vi "Pre Launch Init.vi"(11 "UI in":refnum<class "UI.lvclass">) -> (0 "error out":errorcluster, 3 "UI out":refnum<class "UI.lvclass">)   [LabVIEW 2016, in "UI.lvlib" / "UI.lvclass"]
doc: "Creates user events for the UI actor which later can be used to receive messages"
uses:
  UI.lvclass
  <vilib>/vision/Image Controls.llb/IMAQ Image.ctl
  UI.lvclass/UI.ctl
  <vilib>/ActorFramework/Actor/Actor.lvclass
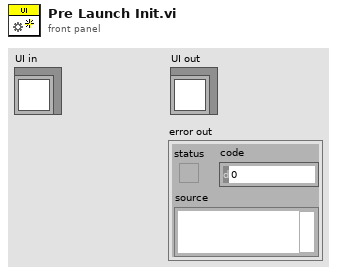
[diagram p1: front panel]
types:
  T1 = typedef "IMAQ Image.ctl" = refnum<image>
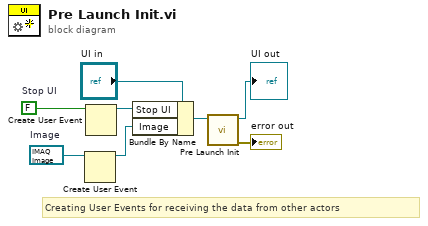
[diagram p0: block diagram]
diagram:
  w2 = T1 refnum  # Image
  w4 = FALSE  # Stop UI
  # "Creating User Events for receiving the data from other actors"
  n1 = Create User Event(user event datatype=w2) -> (user event=w1:refnum<user-event>)  [unwired: 1 in, 1 out]
  n2 = Create User Event(user event datatype=w4) -> (user event=w3:refnum<user-event>)  [unwired: 1 in, 1 out]
  n3 = Bundle By Name(cluster="UI in", "Stop UI"=w3, "Image"=w1) -> (w5:refnum<class "UI.lvclass">)
  n4 = call-parent "Pre Launch Init.vi"("Actor in"=w5) -> ("error out"=→"error out":errorcluster, "Actor out"=→"UI out":refnum<class "UI.lvclass">)  [unwired: 9 in]
